vi "ArrayToExcel.vi"() -> ()   [LabVIEW 2020]
uses:
  <vilib>/Analysis/NI_AALBase.lvlib
panel:
  out "Tabla":string[][](array[string])
  out "Waveform Graph":dbl[][](graph)
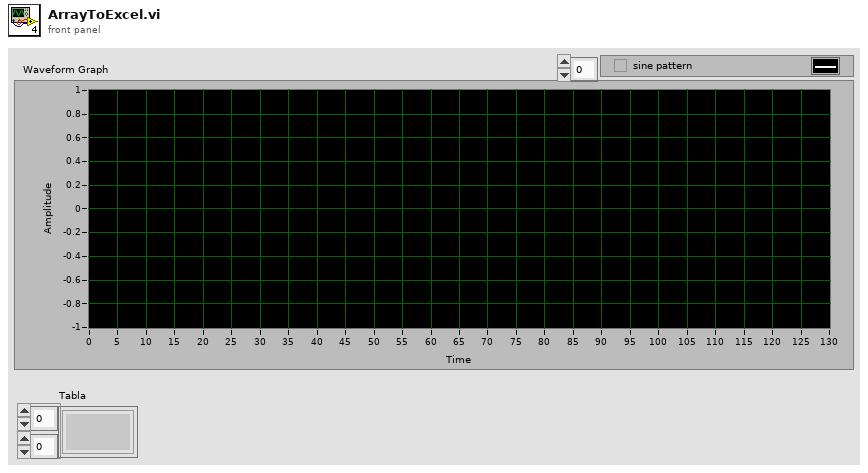
[diagram p1: front panel]
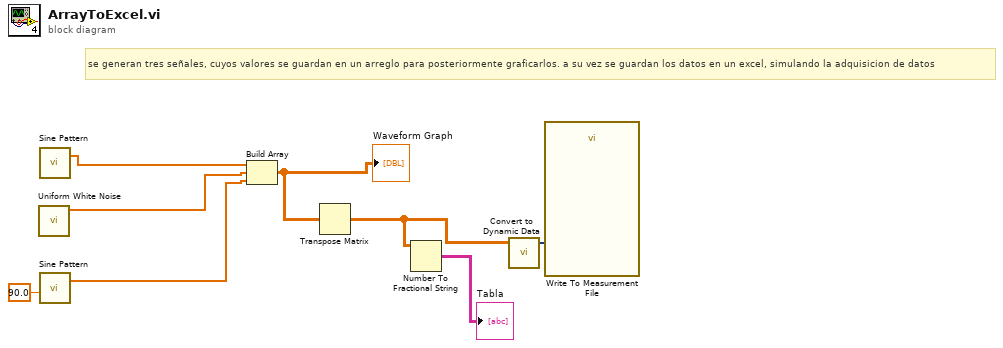
[diagram p0: block diagram]
diagram:
  # "se generan tres señales, cuyos valores se guardan en un arreglo para posteriormente graficarlos. a su vez se guardan los datos en un excel, simulando la adquisicion de datos"
  n1 = call <vilib>:"Uniform White Noise.vi"() -> ("uniform white noise"=w6:dbl[])  [unwired: 10 in, 1 out]
  n2 = call <vilib>:"Sine Pattern.vi"() -> ("Sinusoidal Pattern"=w7:dbl[])  [unwired: 4 in, 1 out]
  n3 = call <vilib>:"Sine Pattern.vi"("phase(degrees)"=90.0) -> ("Sinusoidal Pattern"=w5:dbl[])  [unwired: 3 in, 1 out]
  n4 = Build Array "Build Array"(w7, w6, w5) -> (w4:dbl[][])
  "Waveform Graph" <- w4
  n5 = Transpose Matrix(1:w4) -> (0:w2:dbl[][])
  n6 = Number To Fractional String(number=w2) -> (F-format string=→"Tabla":string[][])  [unwired: 3 in]
  n7 = call "Convert to Dynamic Data"("2D Array"=w2) -> ("Dynamic Data Type"=w1:dynamicdata)  [unwired: 3 in]
  n8 = call "Write To Measurement File"("Signals"=w1) -> ()  [unwired: 16 in, 3 out]
